vi "Manipulator Set XYZ.vi"(8 "error in (no error)":errorcluster, 10 "Coordinates":cluster{"X":i32, "Y":i32, "Z":i32}, 11 "VISA resource in":refnum<visa-resource-name>="COM1") -> (0 "error out":errorcluster, 3 "VISA resource out":refnum<visa-resource-name>)   [LabVIEW 2012, in "Scientifica Manipulator Daemon.lvlib"]
uses:
  Scientifica Manipulator Daemon.lvlib
panel:
  out "Response":string
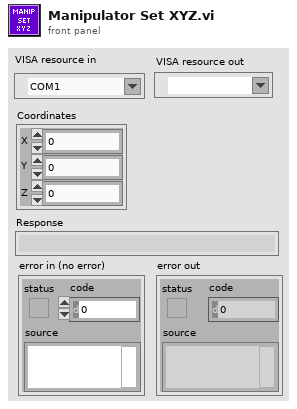
[diagram p1: front panel]
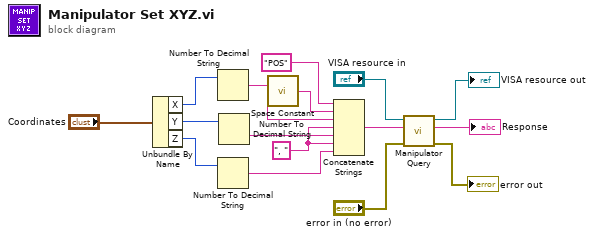
[diagram p0: block diagram]
diagram:
  w10 = ", " ("string")
  n1 = Unbundle By Name("Coordinates") -> ("X"=w4:i32, "Y"=w3:i32, "Z"=w2:i32)
  n2 = Number To Decimal String(number=w4) -> (decimal integer string=w7:string)  [unwired: 1 in]
  n3 = Number To Decimal String(number=w2) -> (decimal integer string=w9:string)  [unwired: 1 in]
  n4 = Number To Decimal String(number=w3) -> (decimal integer string=w8:string)  [unwired: 1 in]
  n5 = call <vilib>:"Space Constant.vi"() -> ("String"=w11:string)
  n6 = Concatenate Strings("POS", w11, w7, w10, w8, w10, w9) -> (w6:string)
  n7 = call "Manipulator Query.vi"("error in (no error)"="error in (no error)", "Command"=w6, "VISA resource in"="VISA resource in") -> ("error out"=→"error out":errorcluster, "Response"=→"Response":string, "VISA resource out"=→"VISA resource out":refnum<visa-resource-name>)  [unwired: 5 in, 1 out]
